vi "Coerce Wheel Angle.vi"(1 "Angle In":dbl) -> (0 "Wheel Angle":dbl)   [LabVIEW 2009]
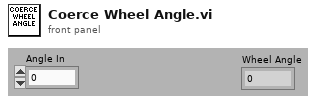
[diagram p1: front panel]
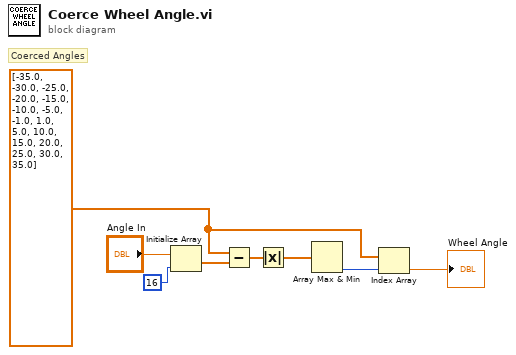
[diagram p0: block diagram]
diagram:
  w2 = dbl[] [-35.0, -30.0, -25.0, -20.0, -15.0, -10.0, -5.0, -1.0, 1.0, 5.0, 10.0, 15.0, 20.0, 25.0, 30.0, 35.0]
  # "Coerced Angles"
  n1 = Initialize Array("Angle In", 16 ("dimension size")) -> (w6:dbl[])
  n2 = Subtract(x=w2, y=w6) -> (x-y=w5:dbl[])
  n3 = Absolute Value(x=w5) -> (abs(x)=w4:dbl[])
  n4 = Array Max & Min(array=w4) -> (min index (indices)=w3:i32)  [unwired: 3 out]
  n5 = Index Array(array=w2, index=w3) -> (element=→"Wheel Angle":dbl)
